vi "Autonomous Independent.vi"() -> ()   [LabVIEW 2017]
doc: "This VI is called when autonomous begins, and will automatically be terminated when autonomous ends. You can carry out timed or sensor driven robot movement independently without needing to return to the caller."
uses:
  <vilib>/Rock Robotics/WPI/Utilities/WPI_GetSetVariantRefNum.vi
  <vilib>/Rock Robotics/Network Tables/NT Write Numeric Array.vi
panel:
  in  "Encoder Input":T1
  out "Rate L 2":dbl
  out "Rate R 2":dbl
  out "Distance L 2":dbl
  out "Direction L 2":bool
  out "Distance R 2":dbl
  out "Direction L 2":bool
  in  "Encoder Input 2":T1
  # "Be sure to right-click and choose Data Operations>>Make Current Value default if you want to save the array values with the VI"
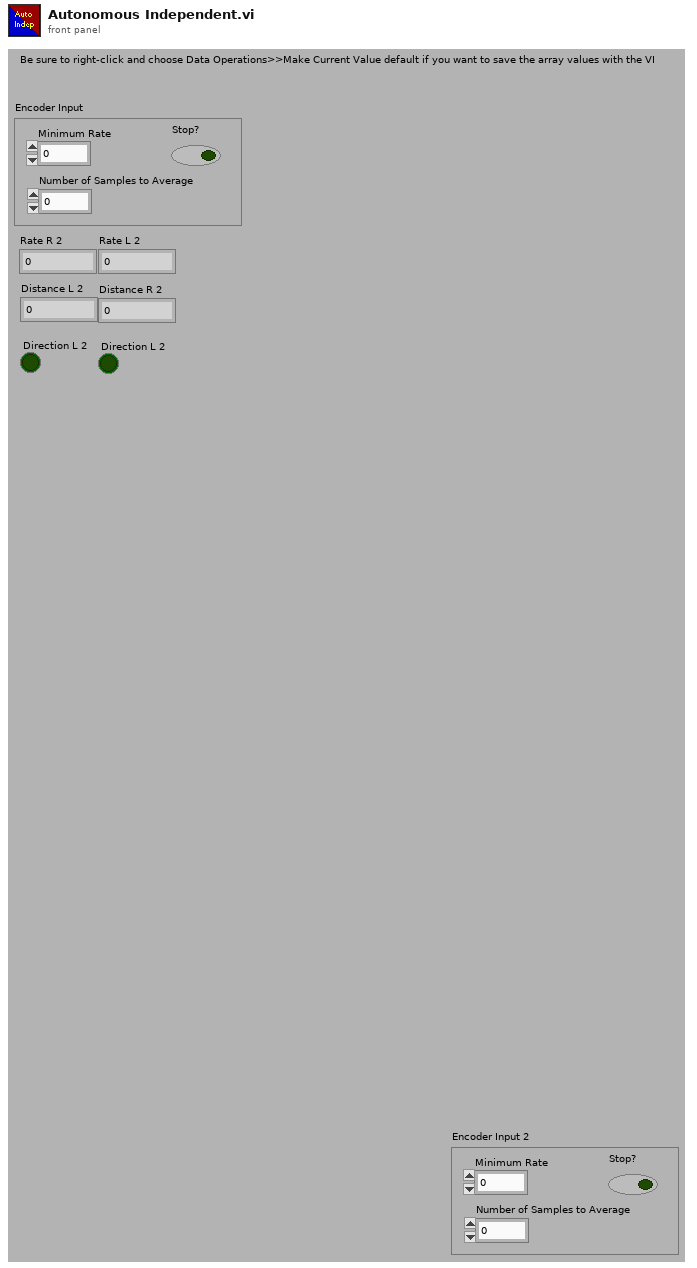
[diagram p1: front panel]
types:
  T1 = cluster{"Minimum Rate":dbl, "Number of Samples to Average":u8, "Stop?":bool}
  T2 = typedef "WPI_JoystickDevRef.ctl" = cluster{"Device":T3}
  T3 = typedef "WPI_JoystickDeviceEnum.ctl" = enum16{"USB 0", "USB 1", "USB 2", "USB 3", "USB 4", "USB 5"}
  T4 = typedef "WPI_RobotDriveDevRef.ctl" = cluster{"DevStatus":errorcluster, "Motors[]":T5[], "Square Inputs":bool, "Max Output":dbl}
  T5 = typedef "WPI_MotorControlDeviceRef.ctl" = cluster{"DeviceStatus":errorcluster, "Type":T6, "PWM":cluster{"PWM Channel":T7, "DeadBand":T8}, "CAN":cluster{"Device Number":u8, "SetOutput VI Ref":variant, "GetOutput VI Ref":variant, "Enable VI Ref":variant, "Disable VI Ref":variant, "Data":variant}, "Invert":bool, "DIO PWM":cluster{"PWM \"Enable\" Channel":T7, "DIOChannel":T9, "PWM Rate":dbl}}
  T6 = typedef "WPI_MotorControlType.ctl" = enum16{"PWM", "CAN", "DIO PWM"}
  T7 = typedef "FPGA_DIOPWMChannel.ctl" = enum8{"PWM 0", "PWM 1", "PWM 2", "PWM 3", "PWM 4", "PWM 5", "PWM 6", "PWM 7", "PWM 8", "PWM 9", "PWM MXP 0", "PWM MXP 1", "PWM MXP 2", "PWM MXP 3", "PWM MXP 4", "PWM MXP 5", "PWM MXP 6", "PWM MXP 7", "PWM MXP 8", "PWM MXP 9", "Invalid"}
  T8 = typedef "WPI_PWMDeadband.ctl" = cluster{"Name":string, "maxPositivePwm":i32, "minPositivePwm":i32, "centerPwm":i32, "maxNegativePwm":i32, "minNegativePwm":i32, "angularRange":u16}
  T9 = typedef "FPGA_DIOChannel.ctl" = enum8{"DIO 0", "DIO 1", "DIO 2", "DIO 3", "DIO 4", "DIO 5", "DIO 6", "DIO 7", "DIO 8", "DIO 9", "DIO MXP 0", "DIO MXP 1", "DIO MXP 2", "DIO MXP 3", "DIO MXP 4", "DIO MXP 5", "DIO MXP 6", "DIO MXP 7", "DIO MXP 8", "DIO MXP 9", "DIO MXP 10", "DIO MXP 11", "DIO MXP 12", "DIO MXP 13", "DIO MXP 14", "DIO MXP 15", "SPI Port CS1", "SPI Port CS2", "SPI Port CS3", "SPI Port MISO", "SPI Port MOSI", "Invalid"}
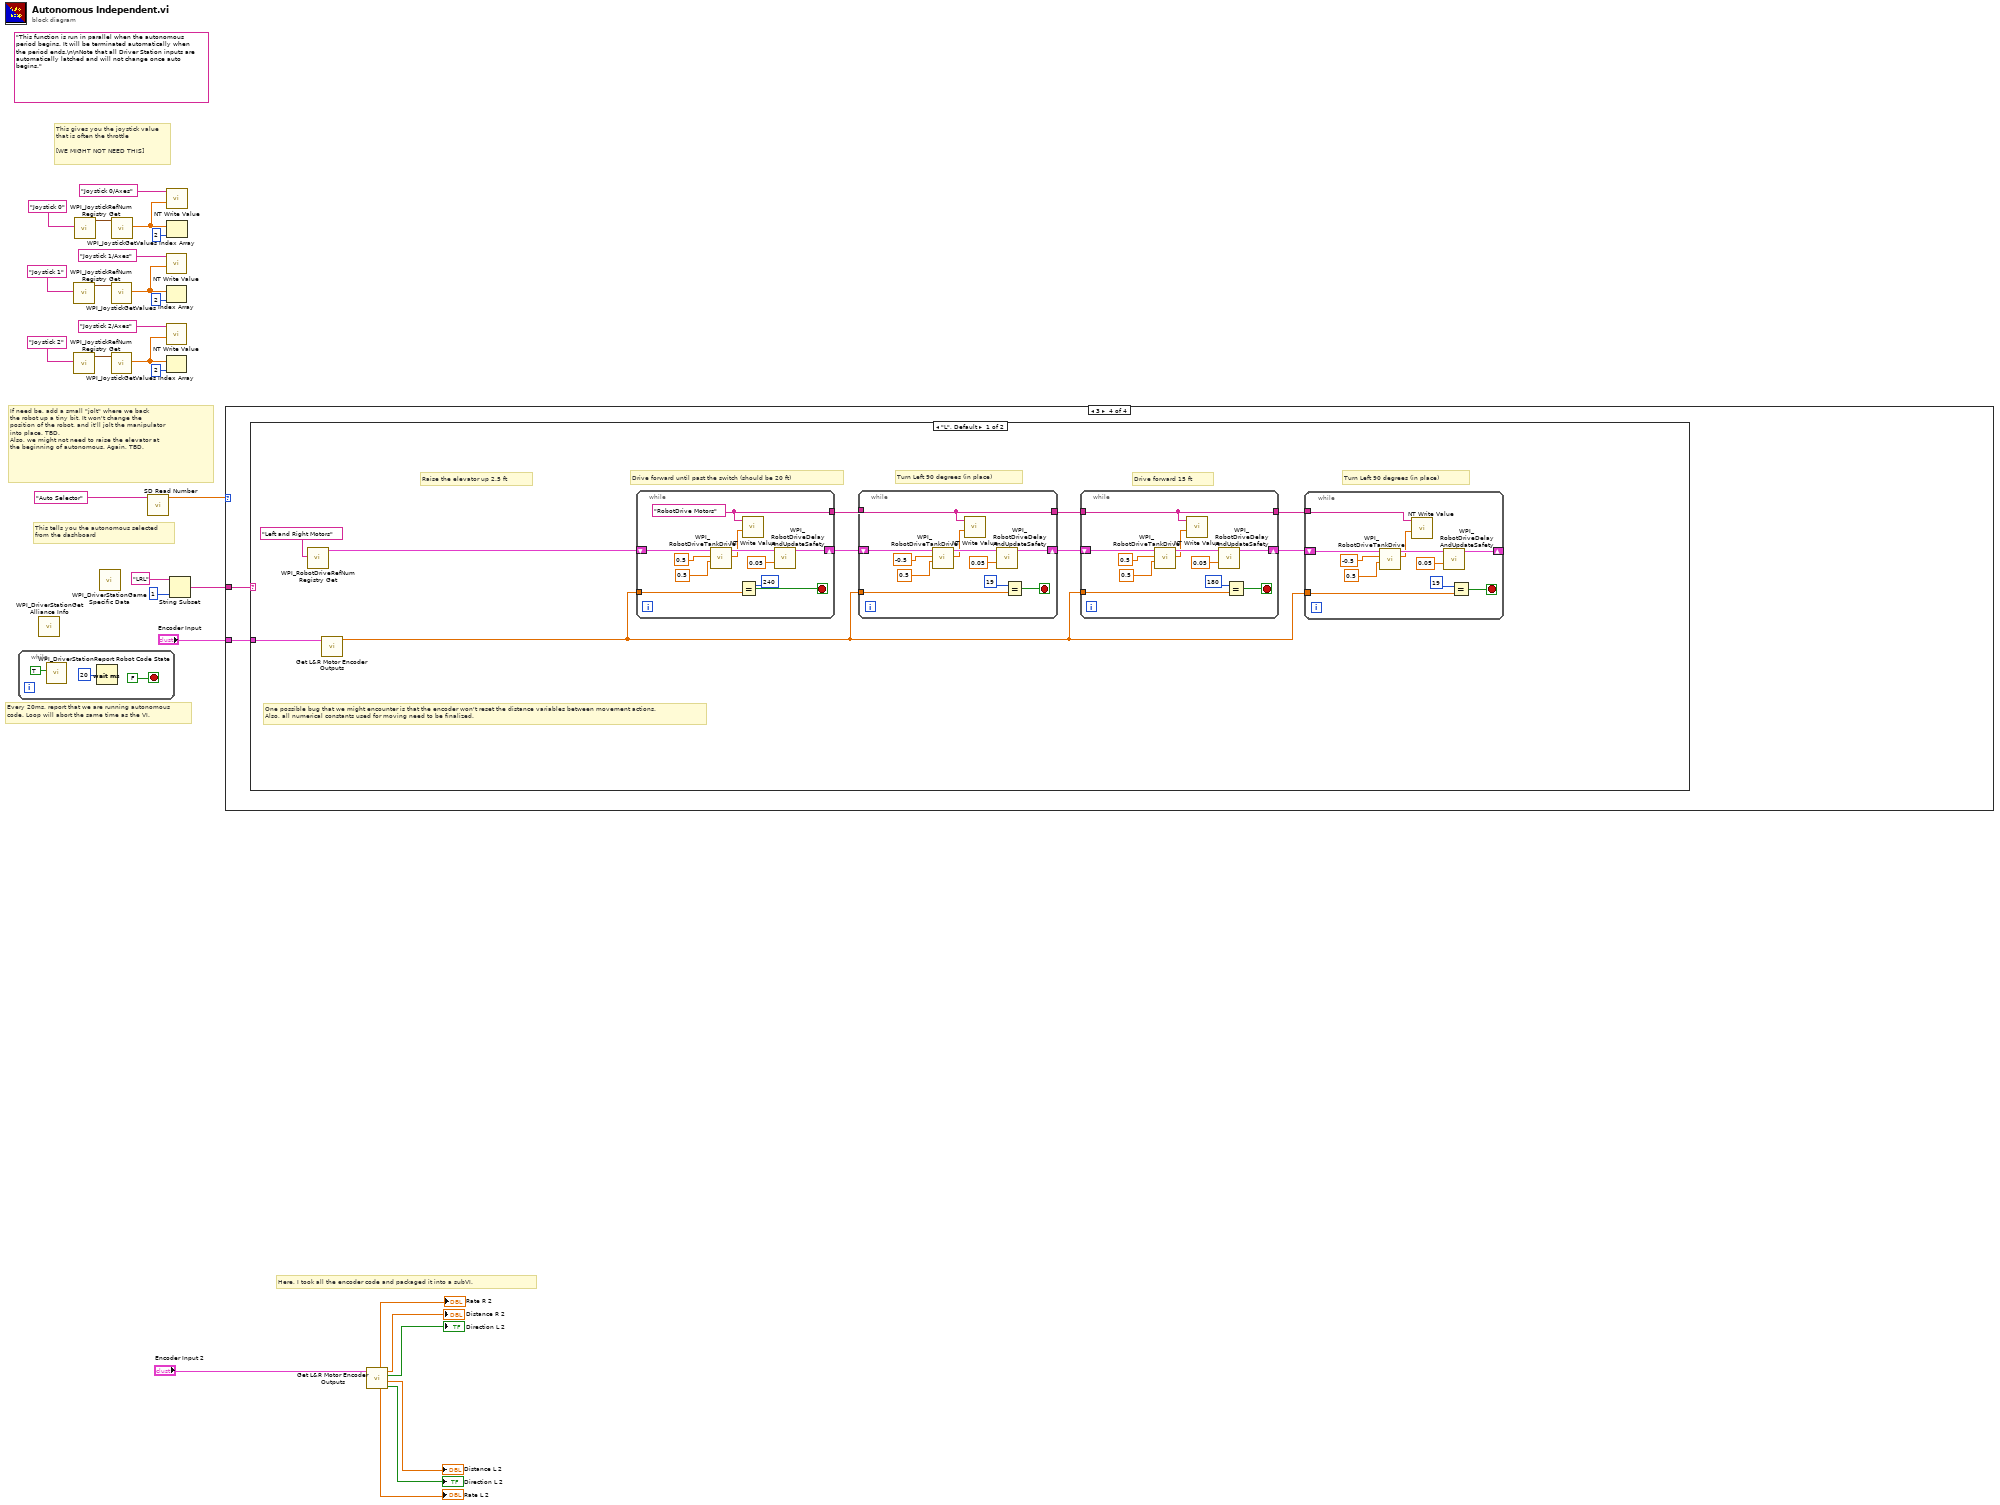
[diagram p0: block diagram]
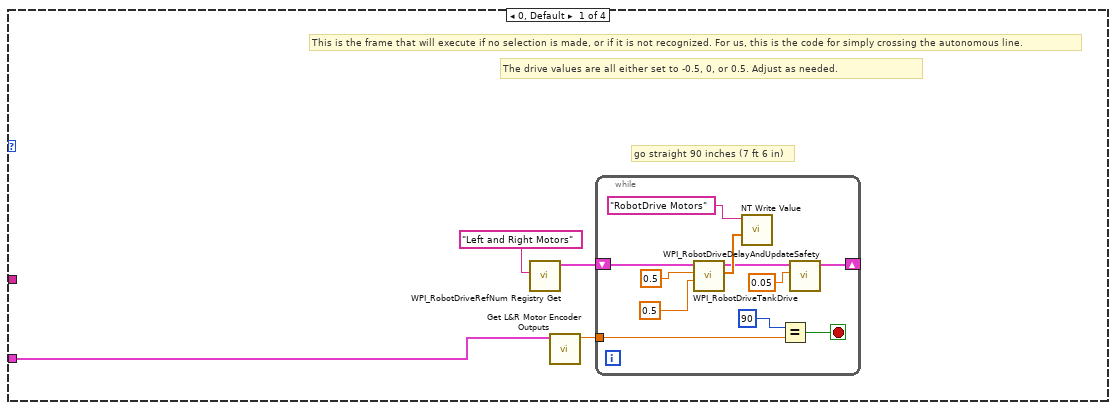
[diagram p2: hidden frame]
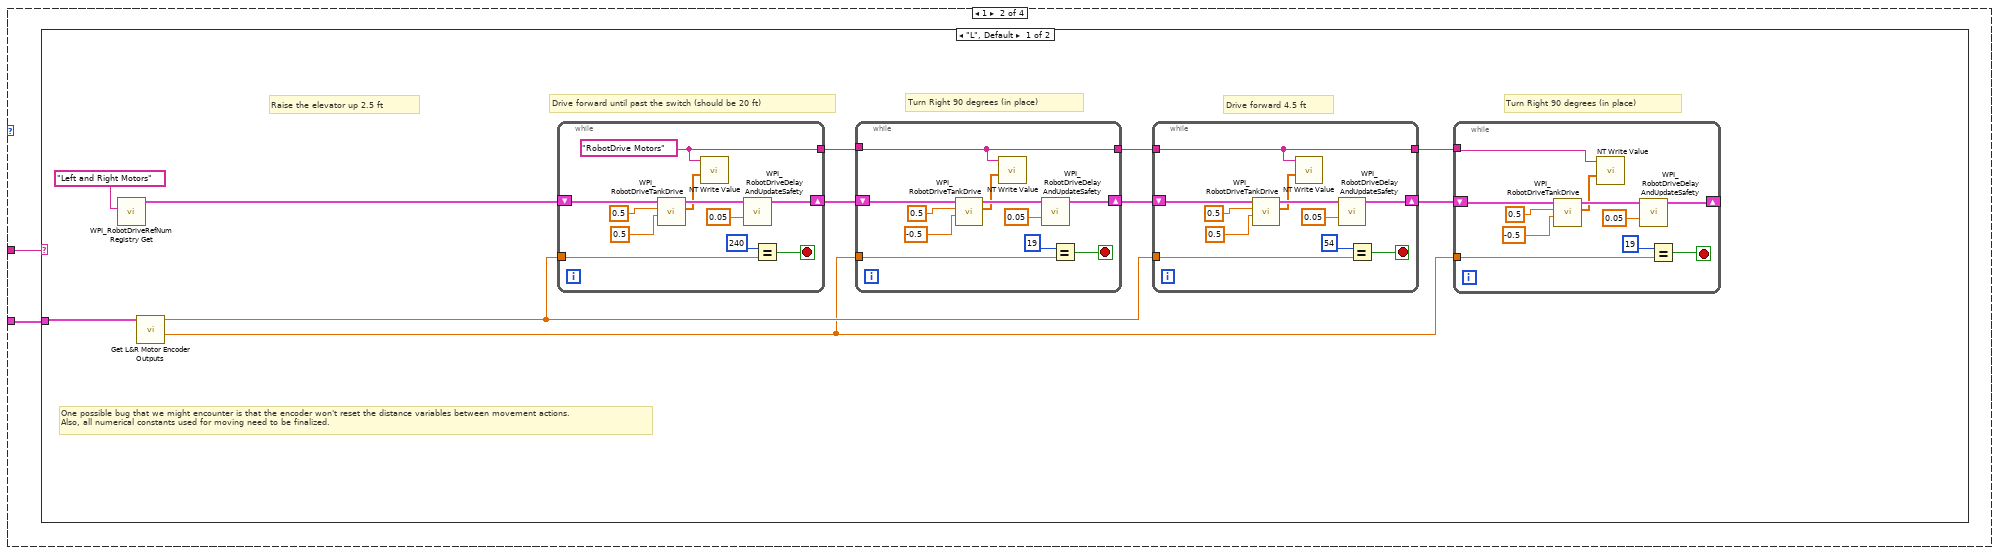
[diagram p3: hidden frame]
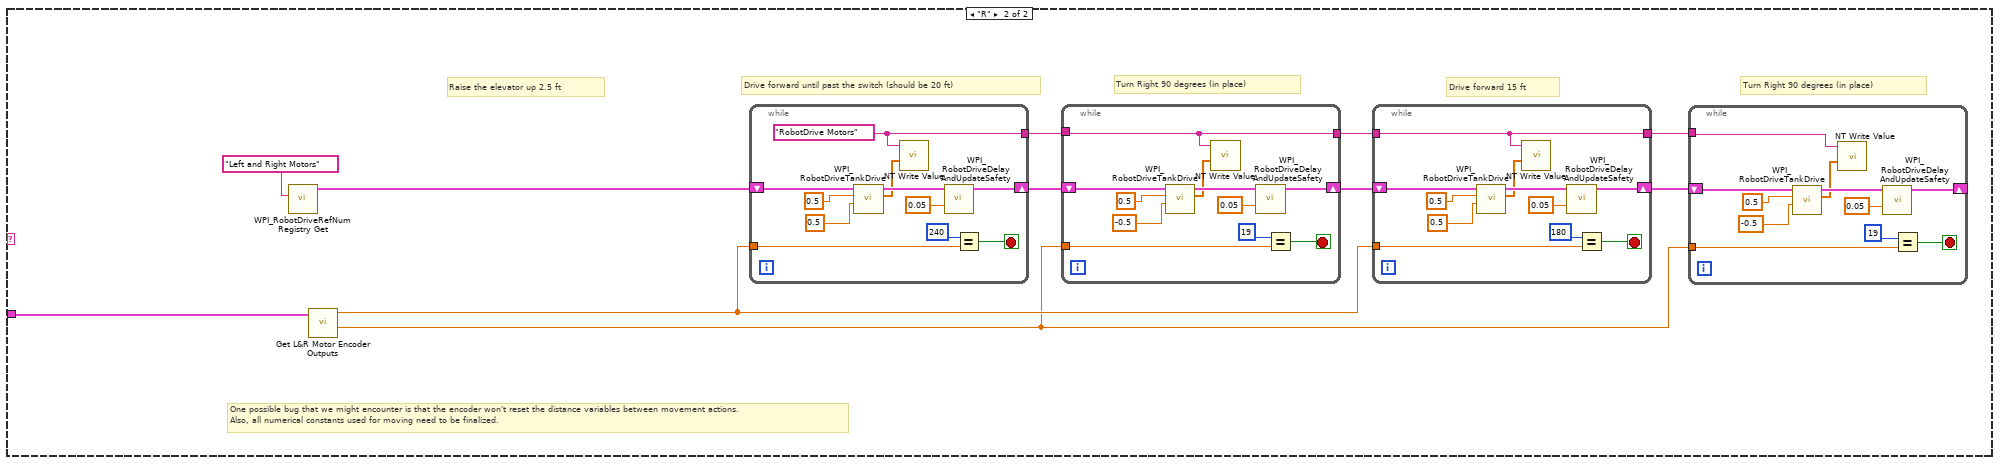
[diagram p4: hidden frame]
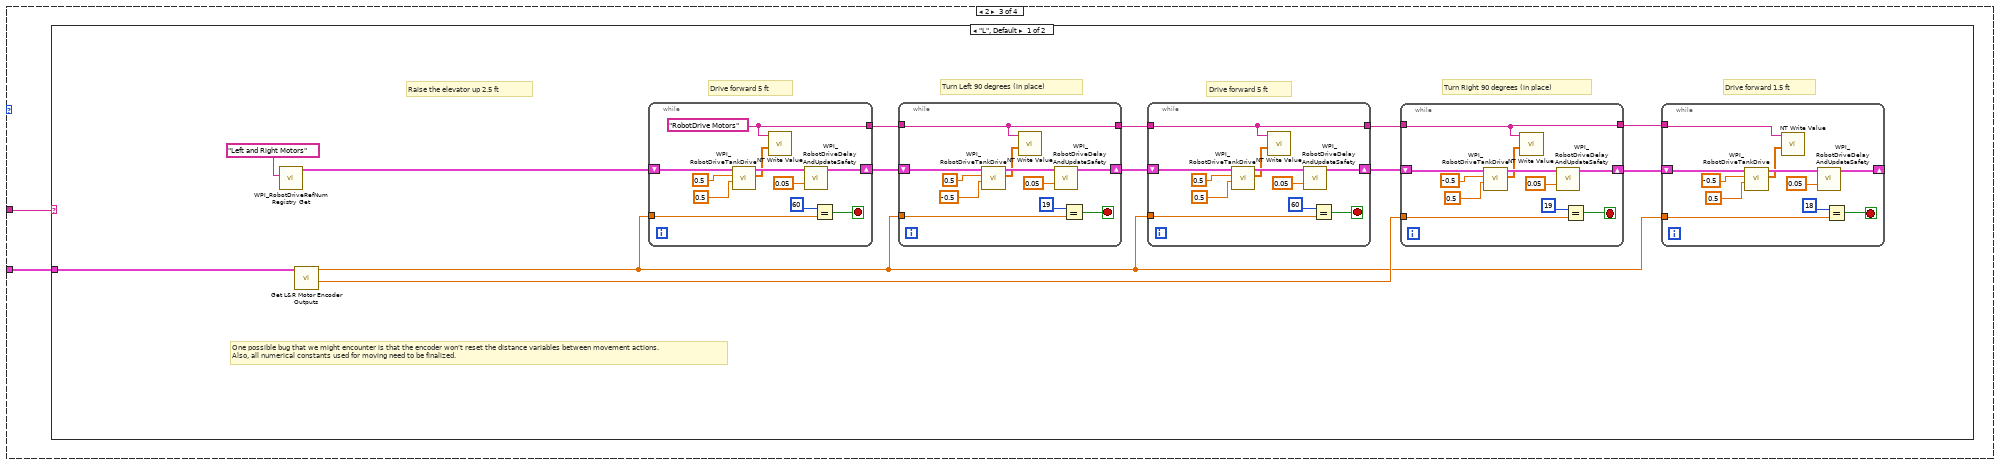
[diagram p5: hidden frame]
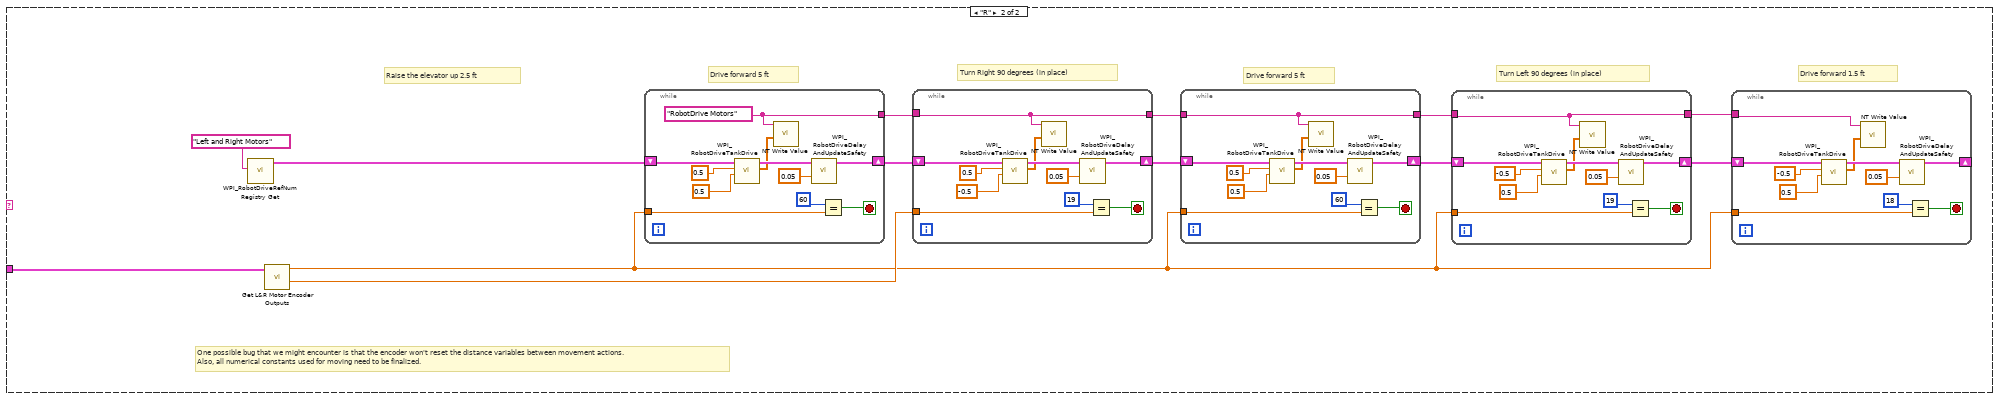
[diagram p6: hidden frame]
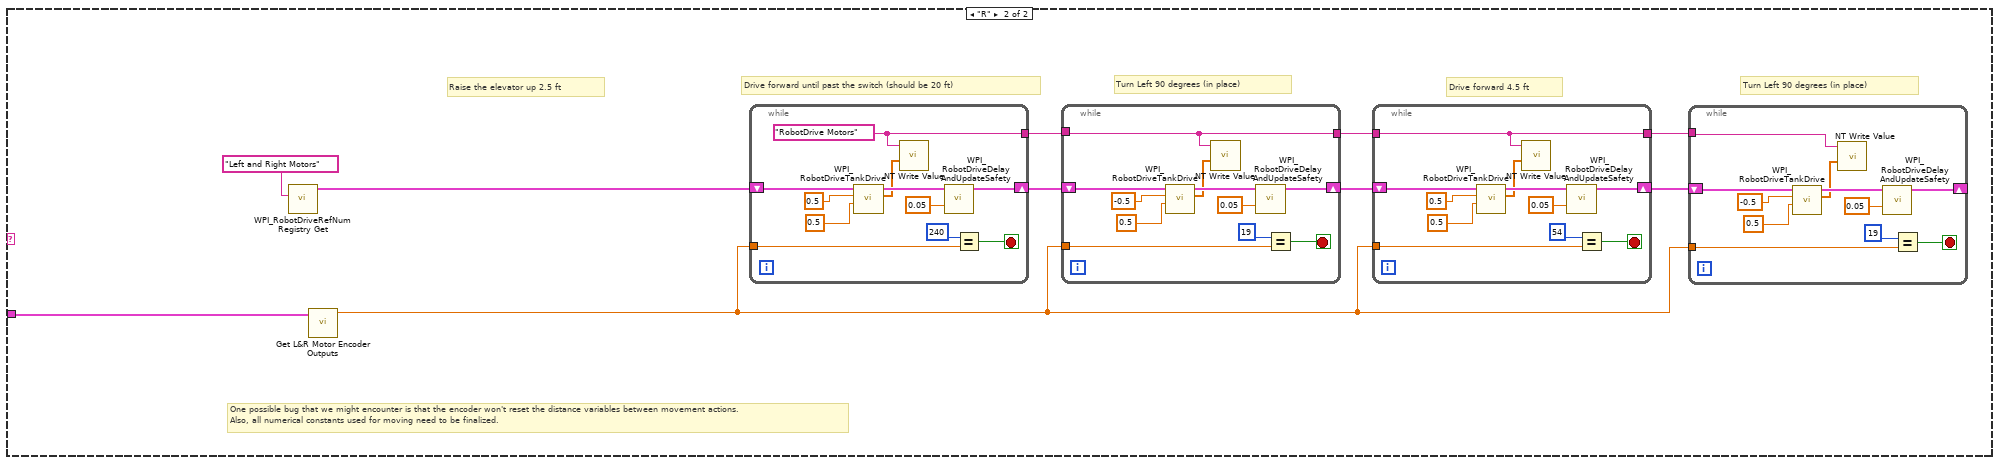
[diagram p7: hidden frame]
diagram:
  (unwired) "This function is run in parallel when the autonomous period begins. It will be terminated automatically when the period ends.\n\nNote that all Driver Station inputs are automatically latched and will not change once auto begins."
  # "If need be, add a small \"jolt\" where we back\nthe robot up a tiny bit. It won't change the\nposition of the robot, and it'll jolt the manipulator\ninto place. TBD.\nAlso, we might not need to raise the elevator at\nthe beginning of autonomous. Again, TBD."
  # "Here, I took all the encoder code and packaged it into a subVI."
  # "This tells you the autonomous selected\nfrom the dashboard"
  # "Every 20ms, report that we are running autonomous\ncode. Loop will abort the same time as the VI."
  # "This gives you the joystick value\nthat is often the throttle\n\n[WE MIGHT NOT NEED THIS]"
  n1 = while {
    stop <- FALSE stop-if-true
    n2 = call <vilib>:"WPI_DriverStationReport Robot Code State.vi"("Autonomous"=TRUE) -> ()  [unwired: 10 in, 1 out]
    n3 = Wait (ms)(milliseconds to wait=u32 20) -> ()  [unwired: 1 out]
  }
  n4 = call <vilib>:"WPI_DriverStationGet Alliance Info.vi"() -> ()  [unwired: 12 out]
  n5 = call <vilib>:"WPI_JoystickRefNum Registry Get.vi"("refnum name"="Joystick 1") -> ("JoystickDevRef"=w22:T2)  [unwired: 1 in, 9 out]
  n6 = call <vilib>:"WPI_JoystickRefNum Registry Get.vi"("refnum name"="Joystick 2") -> ("JoystickDevRef"=w7:T2)  [unwired: 1 in, 9 out]
  n7 = call <vilib>:"WPI_JoystickRefNum Registry Get.vi"("refnum name"="Joystick 0") -> ("JoystickDevRef"=w27:T2)  [unwired: 1 in, 9 out]
  n8 = call <vilib>:"WPI_DriverStationGame Specific Data.vi"() -> ()  [unwired: 11 in, 1 out]
  n9 = call <vilib>:"WPI_JoystickGetValues.vi"("JoystickDevRef"=w22) -> ("Axes"=w20:dbl[])  [unwired: 6 in, 4 out]
  n10 = call <vilib>:"WPI_JoystickGetValues.vi"("JoystickDevRef"=w7) -> ("Axes"=w5:dbl[])  [unwired: 6 in, 4 out]
  n11 = call <vilib>:"WPI_JoystickGetValues.vi"("JoystickDevRef"=w27) -> ("Axes"=w25:dbl[])  [unwired: 6 in, 4 out]
  n12 = call <vilib>:"SD Read Number.vi"("Name"="Auto Selector") -> ("Numeric"=w3:dbl)  [unwired: 8 in, 2 out]
  n13 = call-poly <vilib>:"NT Write Value.vi"("Numeric Array"=w20, "Name"="Joystick 1/Axes") -> ()  [unwired: 9 in, 1 out]
  n14 = Index Array(array=w20, index=2) -> ()  [unwired: 1 out]
  n15 = call-poly <vilib>:"NT Write Value.vi"("Numeric Array"=w5, "Name"="Joystick 2/Axes") -> ()  [unwired: 9 in, 1 out]
  n16 = Index Array(array=w5, index=2) -> ()  [unwired: 1 out]
  n17 = call-poly <vilib>:"NT Write Value.vi"("Numeric Array"=w25, "Name"="Joystick 0/Axes") -> ()  [unwired: 9 in, 1 out]
  n18 = Index Array(array=w25, index=2) -> ()  [unwired: 1 out]
  n19 = String Subset(string="LRL", length (rest)=1) -> (substring=w10:string)  [unwired: 1 in]
  n20 = case shown="3" w3 {
    tunnel: w10 -> [_ w48 w160 w298]
    tunnel: "Encoder Input" -> [w32 w47 w159 w297]
    frame 0, Default {
      # "The drive values are all either set to -0.5, 0, or 0.5. Adjust as needed."
      # "go straight 90 inches (7 ft 6 in)"
      # "This is the frame that will execute if no selection is made, or if it is not recognized. For us, this is the code for simply crossing the autonomous line."
      n21 = call <vilib>:"WPI_RobotDriveRefNum Registry Get.vi"("refnum name"="Left and Right Motors") -> ("RobotDriveDevRef"=w34:T4)  [unwired: 1 in, 9 out]
      n22 = call <vilib>:"Get L&R Motor Encoder Outputs.vi"("Encoder Input in"=w32) -> ("Distance R"=w33:dbl)  [unwired: 5 in, 5 out]
      n23 = while {
        shift-right: [w38] -> _
        shift-left: w34 -> [w43]
        tunnel: w33 -> [w36]
        stop <- w37 stop-if-true
        n24 = call <vilib>:"WPI_RobotDriveTankDrive.vi"("Right axis value"=0.5 ("X axis value"), "Left axis value"=0.5 ("X axis value"), "RobotDriveDevRef"=w43) -> ("Motor Values"=w46:dbl[], "RobotDriveDevRef"=w39:T4)  [unwired: 6 in, 1 out]
        n25 = call-poly <vilib>:"NT Write Value.vi"("Numeric Array"=w46, "Name"="RobotDrive Motors") -> ()  [unwired: 9 in, 1 out]
        n26 = Equal?(x=90, y=w36) -> (x = y?=w37:bool)
        n27 = call <vilib>:"WPI_RobotDriveDelayAndUpdateSafety.vi"("Delay (s)"=0.05, "RobotDriveDevRef"=w39) -> ("RobotDriveDevRef 2"=w38:T4)  [unwired: 8 in, 1 out]
      }
    }
    frame 1 {
      n28 = case shown="\"L\", Default" w48 {
        tunnel: w47 -> [w49 w104]
        frame "L", Default {
          # "Raise the elevator up 2.5 ft"
          # "Turn Right 90 degrees (in place)"
          # "Drive forward 4.5 ft"
          # "One possible bug that we might encounter is that the encoder won't reset the distance variables between movement actions.\nAlso, all numerical constants used for moving need to be finalized."
          # "Turn Right 90 degrees (in place)"
          # "Drive forward until past the switch (should be 20 ft)"
          n29 = call <vilib>:"WPI_RobotDriveRefNum Registry Get.vi"("refnum name"="Left and Right Motors") -> ("RobotDriveDevRef"=w58:T4)  [unwired: 1 in, 9 out]
          n30 = call <vilib>:"Get L&R Motor Encoder Outputs.vi"("Encoder Input in"=w49) -> ("Distance L"=w50:dbl, "Distance R"=w53:dbl)  [unwired: 5 in, 4 out]
          n31 = while {
            tunnel: w53 -> [w102]
            shift-right: [w97] -> w57
            shift-left: w58 -> [w98]
            tunnel: [w96] -> w56
            stop <- w103 stop-if-true
            w96 = "RobotDrive Motors" ("Name")
            n32 = call <vilib>:"WPI_RobotDriveTankDrive.vi"("Right axis value"=0.5 ("X axis value"), "Left axis value"=0.5 ("X axis value"), "RobotDriveDevRef"=w98) -> ("Motor Values"=w100:dbl[], "RobotDriveDevRef"=w101:T4)  [unwired: 6 in, 1 out]
            n33 = call-poly <vilib>:"NT Write Value.vi"("Numeric Array"=w100, "Name"=w96) -> ()  [unwired: 9 in, 1 out]
            n34 = call <vilib>:"WPI_RobotDriveDelayAndUpdateSafety.vi"("Delay (s)"=0.05, "RobotDriveDevRef"=w101) -> ("RobotDriveDevRef 2"=w97:T4)  [unwired: 8 in, 1 out]
            n35 = Equal?(x=240, y=w102) -> (x = y?=w103:bool)
          }
          n36 = while {
            shift-right: [w87] -> w54
            shift-left: w57 -> [w88]
            tunnel: [w83] -> w55
            tunnel: w56 -> [w83]
            tunnel: w50 -> [w82]
            stop <- w92 stop-if-true
            n37 = call <vilib>:"WPI_RobotDriveTankDrive.vi"("Right axis value"=-0.5 ("X axis value"), "Left axis value"=0.5 ("X axis value"), "RobotDriveDevRef"=w88) -> ("Motor Values"=w90:dbl[], "RobotDriveDevRef"=w91:T4)  [unwired: 6 in, 1 out]
            n38 = call-poly <vilib>:"NT Write Value.vi"("Numeric Array"=w90, "Name"=w83) -> ()  [unwired: 9 in, 1 out]
            n39 = call <vilib>:"WPI_RobotDriveDelayAndUpdateSafety.vi"("Delay (s)"=0.05, "RobotDriveDevRef"=w91) -> ("RobotDriveDevRef 2"=w87:T4)  [unwired: 8 in, 1 out]
            n40 = Equal?(x=19, y=w82) -> (x = y?=w92:bool)
          }
          n41 = while {
            tunnel: w53 -> [w80]
            shift-right: [w75] -> w51
            shift-left: w54 -> [w76]
            tunnel: [w71] -> w52
            tunnel: w55 -> [w71]
            stop <- w81 stop-if-true
            n42 = call <vilib>:"WPI_RobotDriveTankDrive.vi"("Right axis value"=0.5 ("X axis value"), "Left axis value"=0.5 ("X axis value"), "RobotDriveDevRef"=w76) -> ("Motor Values"=w78:dbl[], "RobotDriveDevRef"=w79:T4)  [unwired: 6 in, 1 out]
            n43 = call-poly <vilib>:"NT Write Value.vi"("Numeric Array"=w78, "Name"=w71) -> ()  [unwired: 9 in, 1 out]
            n44 = call <vilib>:"WPI_RobotDriveDelayAndUpdateSafety.vi"("Delay (s)"=0.05, "RobotDriveDevRef"=w79) -> ("RobotDriveDevRef 2"=w75:T4)  [unwired: 8 in, 1 out]
            n45 = Equal?(x=54, y=w80) -> (x = y?=w81:bool)
          }
          n46 = while {
            shift-right: [w65] -> _
            shift-left: w51 -> [w66]
            tunnel: w52 -> [w61]
            tunnel: w50 -> [w60]
            stop <- w70 stop-if-true
            n47 = call <vilib>:"WPI_RobotDriveTankDrive.vi"("Right axis value"=-0.5 ("X axis value"), "Left axis value"=0.5 ("X axis value"), "RobotDriveDevRef"=w66) -> ("Motor Values"=w68:dbl[], "RobotDriveDevRef"=w69:T4)  [unwired: 6 in, 1 out]
            n48 = call-poly <vilib>:"NT Write Value.vi"("Numeric Array"=w68, "Name"=w61) -> ()  [unwired: 9 in, 1 out]
            n49 = call <vilib>:"WPI_RobotDriveDelayAndUpdateSafety.vi"("Delay (s)"=0.05, "RobotDriveDevRef"=w69) -> ("RobotDriveDevRef 2"=w65:T4)  [unwired: 8 in, 1 out]
            n50 = Equal?(x=19, y=w60) -> (x = y?=w70:bool)
          }
        }
        frame "R" {
          # "Raise the elevator up 2.5 ft"
          # "Turn Right 90 degrees (in place)"
          # "Drive forward 15 ft"
          # "One possible bug that we might encounter is that the encoder won't reset the distance variables between movement actions.\nAlso, all numerical constants used for moving need to be finalized."
          # "Turn Right 90 degrees (in place)"
          # "Drive forward until past the switch (should be 20 ft)"
          n51 = call <vilib>:"WPI_RobotDriveRefNum Registry Get.vi"("refnum name"="Left and Right Motors") -> ("RobotDriveDevRef"=w113:T4)  [unwired: 1 in, 9 out]
          n52 = call <vilib>:"Get L&R Motor Encoder Outputs.vi"("Encoder Input in"=w104) -> ("Distance L"=w105:dbl, "Distance R"=w108:dbl)  [unwired: 5 in, 4 out]
          n53 = while {
            tunnel: w108 -> [w157]
            shift-right: [w152] -> w112
            shift-left: w113 -> [w153]
            tunnel: [w151] -> w111
            stop <- w158 stop-if-true
            w151 = "RobotDrive Motors" ("Name")
            n54 = call <vilib>:"WPI_RobotDriveTankDrive.vi"("Right axis value"=0.5 ("X axis value"), "Left axis value"=0.5 ("X axis value"), "RobotDriveDevRef"=w153) -> ("Motor Values"=w155:dbl[], "RobotDriveDevRef"=w156:T4)  [unwired: 6 in, 1 out]
            n55 = call-poly <vilib>:"NT Write Value.vi"("Numeric Array"=w155, "Name"=w151) -> ()  [unwired: 9 in, 1 out]
            n56 = call <vilib>:"WPI_RobotDriveDelayAndUpdateSafety.vi"("Delay (s)"=0.05, "RobotDriveDevRef"=w156) -> ("RobotDriveDevRef 2"=w152:T4)  [unwired: 8 in, 1 out]
            n57 = Equal?(x=240, y=w157) -> (x = y?=w158:bool)
          }
          n58 = while {
            shift-right: [w142] -> w109
            shift-left: w112 -> [w143]
            tunnel: [w138] -> w110
            tunnel: w111 -> [w138]
            tunnel: w105 -> [w137]
            stop <- w147 stop-if-true
            n59 = call <vilib>:"WPI_RobotDriveTankDrive.vi"("Right axis value"=-0.5 ("X axis value"), "Left axis value"=0.5 ("X axis value"), "RobotDriveDevRef"=w143) -> ("Motor Values"=w145:dbl[], "RobotDriveDevRef"=w146:T4)  [unwired: 6 in, 1 out]
            n60 = call-poly <vilib>:"NT Write Value.vi"("Numeric Array"=w145, "Name"=w138) -> ()  [unwired: 9 in, 1 out]
            n61 = call <vilib>:"WPI_RobotDriveDelayAndUpdateSafety.vi"("Delay (s)"=0.05, "RobotDriveDevRef"=w146) -> ("RobotDriveDevRef 2"=w142:T4)  [unwired: 8 in, 1 out]
            n62 = Equal?(x=19, y=w137) -> (x = y?=w147:bool)
          }
          n63 = while {
            tunnel: w108 -> [w135]
            shift-right: [w130] -> w106
            shift-left: w109 -> [w131]
            tunnel: [w126] -> w107
            tunnel: w110 -> [w126]
            stop <- w136 stop-if-true
            n64 = call <vilib>:"WPI_RobotDriveTankDrive.vi"("Right axis value"=0.5 ("X axis value"), "Left axis value"=0.5 ("X axis value"), "RobotDriveDevRef"=w131) -> ("Motor Values"=w133:dbl[], "RobotDriveDevRef"=w134:T4)  [unwired: 6 in, 1 out]
            n65 = call-poly <vilib>:"NT Write Value.vi"("Numeric Array"=w133, "Name"=w126) -> ()  [unwired: 9 in, 1 out]
            n66 = call <vilib>:"WPI_RobotDriveDelayAndUpdateSafety.vi"("Delay (s)"=0.05, "RobotDriveDevRef"=w134) -> ("RobotDriveDevRef 2"=w130:T4)  [unwired: 8 in, 1 out]
            n67 = Equal?(x=180, y=w135) -> (x = y?=w136:bool)
          }
          n68 = while {
            shift-right: [w120] -> _
            shift-left: w106 -> [w121]
            tunnel: w107 -> [w116]
            tunnel: w105 -> [w115]
            stop <- w125 stop-if-true
            n69 = call <vilib>:"WPI_RobotDriveTankDrive.vi"("Right axis value"=-0.5 ("X axis value"), "Left axis value"=0.5 ("X axis value"), "RobotDriveDevRef"=w121) -> ("Motor Values"=w123:dbl[], "RobotDriveDevRef"=w124:T4)  [unwired: 6 in, 1 out]
            n70 = call-poly <vilib>:"NT Write Value.vi"("Numeric Array"=w123, "Name"=w116) -> ()  [unwired: 9 in, 1 out]
            n71 = call <vilib>:"WPI_RobotDriveDelayAndUpdateSafety.vi"("Delay (s)"=0.05, "RobotDriveDevRef"=w124) -> ("RobotDriveDevRef 2"=w120:T4)  [unwired: 8 in, 1 out]
            n72 = Equal?(x=19, y=w115) -> (x = y?=w125:bool)
          }
        }
      }
    }
    frame 2 {
      n73 = case shown="\"L\", Default" w160 {
        tunnel: w159 -> [w163 w232]
        frame "L", Default {
          # "Drive forward 1.5 ft"
          # "Raise the elevator up 2.5 ft"
          # "Turn Right 90 degrees (in place)"
          # "Drive forward 5 ft"
          # "One possible bug that we might encounter is that the encoder won't reset the distance variables between movement actions.\nAlso, all numerical constants used for moving need to be finalized."
          # "Turn Left 90 degrees (in place)"
          # "Drive forward 5 ft"
          n74 = call <vilib>:"WPI_RobotDriveRefNum Registry Get.vi"("refnum name"="Left and Right Motors") -> ("RobotDriveDevRef"=w165:T4)  [unwired: 1 in, 9 out]
          n75 = call <vilib>:"Get L&R Motor Encoder Outputs.vi"("Encoder Input in"=w163) -> ("Distance L"=w162:dbl, "Distance R"=w161:dbl)  [unwired: 5 in, 4 out]
          n76 = while {
            tunnel: w161 -> [w227]
            shift-right: [w222] -> w166
            shift-left: w165 -> [w223]
            tunnel: [w221] -> w167
            stop <- w228 stop-if-true
            w221 = "RobotDrive Motors" ("Name")
            n77 = call <vilib>:"WPI_RobotDriveTankDrive.vi"("Right axis value"=0.5 ("X axis value"), "Left axis value"=0.5 ("X axis value"), "RobotDriveDevRef"=w223) -> ("Motor Values"=w225:dbl[], "RobotDriveDevRef"=w226:T4)  [unwired: 6 in, 1 out]
            n78 = call-poly <vilib>:"NT Write Value.vi"("Numeric Array"=w225, "Name"=w221) -> ()  [unwired: 9 in, 1 out]
            n79 = call <vilib>:"WPI_RobotDriveDelayAndUpdateSafety.vi"("Delay (s)"=0.05, "RobotDriveDevRef"=w226) -> ("RobotDriveDevRef 2"=w222:T4)  [unwired: 8 in, 1 out]
            n80 = Equal?(x=60, y=w227) -> (x = y?=w228:bool)
          }
          n81 = while {
            shift-right: [w212] -> w169
            shift-left: w166 -> [w213]
            tunnel: [w208] -> w168
            tunnel: w167 -> [w208]
            tunnel: w161 -> [w207]
            stop <- w217 stop-if-true
            n82 = call <vilib>:"WPI_RobotDriveTankDrive.vi"("Right axis value"=-0.5 ("X axis value"), "Left axis value"=0.5 ("X axis value"), "RobotDriveDevRef"=w213) -> ("Motor Values"=w215:dbl[], "RobotDriveDevRef"=w216:T4)  [unwired: 6 in, 1 out]
            n83 = call-poly <vilib>:"NT Write Value.vi"("Numeric Array"=w215, "Name"=w208) -> ()  [unwired: 9 in, 1 out]
            n84 = call <vilib>:"WPI_RobotDriveDelayAndUpdateSafety.vi"("Delay (s)"=0.05, "RobotDriveDevRef"=w216) -> ("RobotDriveDevRef 2"=w212:T4)  [unwired: 8 in, 1 out]
            n85 = Equal?(x=19, y=w207) -> (x = y?=w217:bool)
          }
          n86 = while {
            tunnel: w161 -> [w205]
            shift-right: [w200] -> w171
            shift-left: w169 -> [w201]
            tunnel: [w196] -> w170
            tunnel: w168 -> [w196]
            stop <- w206 stop-if-true
            n87 = call <vilib>:"WPI_RobotDriveTankDrive.vi"("Right axis value"=0.5 ("X axis value"), "Left axis value"=0.5 ("X axis value"), "RobotDriveDevRef"=w201) -> ("Motor Values"=w203:dbl[], "RobotDriveDevRef"=w204:T4)  [unwired: 6 in, 1 out]
            n88 = call-poly <vilib>:"NT Write Value.vi"("Numeric Array"=w203, "Name"=w196) -> ()  [unwired: 9 in, 1 out]
            n89 = call <vilib>:"WPI_RobotDriveDelayAndUpdateSafety.vi"("Delay (s)"=0.05, "RobotDriveDevRef"=w204) -> ("RobotDriveDevRef 2"=w200:T4)  [unwired: 8 in, 1 out]
            n90 = Equal?(x=60, y=w205) -> (x = y?=w206:bool)
          }
          n91 = while {
            shift-right: [w190] -> w172
            shift-left: w171 -> [w191]
            tunnel: w170 -> [w185]
            tunnel: w162 -> [w186]
            tunnel: [w185] -> w173
            stop <- w195 stop-if-true
            n92 = call <vilib>:"WPI_RobotDriveTankDrive.vi"("Right axis value"=0.5 ("X axis value"), "Left axis value"=-0.5 ("X axis value"), "RobotDriveDevRef"=w191) -> ("Motor Values"=w193:dbl[], "RobotDriveDevRef"=w194:T4)  [unwired: 6 in, 1 out]
            n93 = call-poly <vilib>:"NT Write Value.vi"("Numeric Array"=w193, "Name"=w185) -> ()  [unwired: 9 in, 1 out]
            n94 = call <vilib>:"WPI_RobotDriveDelayAndUpdateSafety.vi"("Delay (s)"=0.05, "RobotDriveDevRef"=w194) -> ("RobotDriveDevRef 2"=w190:T4)  [unwired: 8 in, 1 out]
            n95 = Equal?(x=19, y=w186) -> (x = y?=w195:bool)
          }
          n96 = while {
            shift-right: [w179] -> _
            shift-left: w172 -> [w180]
            tunnel: w173 -> [w175]
            tunnel: w161 -> [w174]
            stop <- w184 stop-if-true
            n97 = call <vilib>:"WPI_RobotDriveTankDrive.vi"("Right axis value"=0.5 ("X axis value"), "Left axis value"=-0.5 ("X axis value"), "RobotDriveDevRef"=w180) -> ("Motor Values"=w182:dbl[], "RobotDriveDevRef"=w183:T4)  [unwired: 6 in, 1 out]
            n98 = call-poly <vilib>:"NT Write Value.vi"("Numeric Array"=w182, "Name"=w175) -> ()  [unwired: 9 in, 1 out]
            n99 = call <vilib>:"WPI_RobotDriveDelayAndUpdateSafety.vi"("Delay (s)"=0.05, "RobotDriveDevRef"=w183) -> ("RobotDriveDevRef 2"=w179:T4)  [unwired: 8 in, 1 out]
            n100 = Equal?(x=18, y=w174) -> (x = y?=w184:bool)
          }
        }
        frame "R" {
          # "Drive forward 1.5 ft"
          # "Raise the elevator up 2.5 ft"
          # "Turn Left 90 degrees (in place)"
          # "Drive forward 5 ft"
          # "One possible bug that we might encounter is that the encoder won't reset the distance variables between movement actions.\nAlso, all numerical constants used for moving need to be finalized."
          # "Turn Right 90 degrees (in place)"
          # "Drive forward 5 ft"
          n101 = call <vilib>:"WPI_RobotDriveRefNum Registry Get.vi"("refnum name"="Left and Right Motors") -> ("RobotDriveDevRef"=w240:T4)  [unwired: 1 in, 9 out]
          n102 = call <vilib>:"Get L&R Motor Encoder Outputs.vi"("Encoder Input in"=w232) -> ("Distance L"=w233:dbl, "Distance R"=w229:dbl)  [unwired: 5 in, 4 out]
          n103 = while {
            tunnel: w229 -> [w295]
            shift-right: [w290] -> w239
            shift-left: w240 -> [w291]
            tunnel: [w289] -> w238
            stop <- w296 stop-if-true
            w289 = "RobotDrive Motors" ("Name")
            n104 = call <vilib>:"WPI_RobotDriveTankDrive.vi"("Right axis value"=0.5 ("X axis value"), "Left axis value"=0.5 ("X axis value"), "RobotDriveDevRef"=w291) -> ("Motor Values"=w293:dbl[], "RobotDriveDevRef"=w294:T4)  [unwired: 6 in, 1 out]
            n105 = call-poly <vilib>:"NT Write Value.vi"("Numeric Array"=w293, "Name"=w289) -> ()  [unwired: 9 in, 1 out]
            n106 = call <vilib>:"WPI_RobotDriveDelayAndUpdateSafety.vi"("Delay (s)"=0.05, "RobotDriveDevRef"=w294) -> ("RobotDriveDevRef 2"=w290:T4)  [unwired: 8 in, 1 out]
            n107 = Equal?(x=60, y=w295) -> (x = y?=w296:bool)
          }
          n108 = while {
            shift-right: [w280] -> w236
            shift-left: w239 -> [w281]
            tunnel: [w276] -> w237
            tunnel: w238 -> [w276]
            tunnel: w233 -> [w275]
            stop <- w285 stop-if-true
            n109 = call <vilib>:"WPI_RobotDriveTankDrive.vi"("Right axis value"=-0.5 ("X axis value"), "Left axis value"=0.5 ("X axis value"), "RobotDriveDevRef"=w281) -> ("Motor Values"=w283:dbl[], "RobotDriveDevRef"=w284:T4)  [unwired: 6 in, 1 out]
            n110 = call-poly <vilib>:"NT Write Value.vi"("Numeric Array"=w283, "Name"=w276) -> ()  [unwired: 9 in, 1 out]
            n111 = call <vilib>:"WPI_RobotDriveDelayAndUpdateSafety.vi"("Delay (s)"=0.05, "RobotDriveDevRef"=w284) -> ("RobotDriveDevRef 2"=w280:T4)  [unwired: 8 in, 1 out]
            n112 = Equal?(x=19, y=w275) -> (x = y?=w285:bool)
          }
          n113 = while {
            tunnel: w229 -> [w273]
            shift-right: [w268] -> w234
            shift-left: w236 -> [w269]
            tunnel: [w264] -> w235
            tunnel: w237 -> [w264]
            stop <- w274 stop-if-true
            n114 = call <vilib>:"WPI_RobotDriveTankDrive.vi"("Right axis value"=0.5 ("X axis value"), "Left axis value"=0.5 ("X axis value"), "RobotDriveDevRef"=w269) -> ("Motor Values"=w271:dbl[], "RobotDriveDevRef"=w272:T4)  [unwired: 6 in, 1 out]
            n115 = call-poly <vilib>:"NT Write Value.vi"("Numeric Array"=w271, "Name"=w264) -> ()  [unwired: 9 in, 1 out]
            n116 = call <vilib>:"WPI_RobotDriveDelayAndUpdateSafety.vi"("Delay (s)"=0.05, "RobotDriveDevRef"=w272) -> ("RobotDriveDevRef 2"=w268:T4)  [unwired: 8 in, 1 out]
            n117 = Equal?(x=60, y=w273) -> (x = y?=w274:bool)
          }
          n118 = while {
            shift-right: [w258] -> w231
            shift-left: w234 -> [w259]
            tunnel: w235 -> [w253]
            tunnel: w229 -> [w254]
            tunnel: [w253] -> w230
            stop <- w263 stop-if-true
            n119 = call <vilib>:"WPI_RobotDriveTankDrive.vi"("Right axis value"=0.5 ("X axis value"), "Left axis value"=-0.5 ("X axis value"), "RobotDriveDevRef"=w259) -> ("Motor Values"=w261:dbl[], "RobotDriveDevRef"=w262:T4)  [unwired: 6 in, 1 out]
            n120 = call-poly <vilib>:"NT Write Value.vi"("Numeric Array"=w261, "Name"=w253) -> ()  [unwired: 9 in, 1 out]
            n121 = call <vilib>:"WPI_RobotDriveDelayAndUpdateSafety.vi"("Delay (s)"=0.05, "RobotDriveDevRef"=w262) -> ("RobotDriveDevRef 2"=w258:T4)  [unwired: 8 in, 1 out]
            n122 = Equal?(x=19, y=w254) -> (x = y?=w263:bool)
          }
          n123 = while {
            shift-right: [w247] -> _
            shift-left: w231 -> [w248]
            tunnel: w230 -> [w243]
            tunnel: w229 -> [w242]
            stop <- w252 stop-if-true
            n124 = call <vilib>:"WPI_RobotDriveTankDrive.vi"("Right axis value"=0.5 ("X axis value"), "Left axis value"=-0.5 ("X axis value"), "RobotDriveDevRef"=w248) -> ("Motor Values"=w250:dbl[], "RobotDriveDevRef"=w251:T4)  [unwired: 6 in, 1 out]
            n125 = call-poly <vilib>:"NT Write Value.vi"("Numeric Array"=w250, "Name"=w243) -> ()  [unwired: 9 in, 1 out]
            n126 = call <vilib>:"WPI_RobotDriveDelayAndUpdateSafety.vi"("Delay (s)"=0.05, "RobotDriveDevRef"=w251) -> ("RobotDriveDevRef 2"=w247:T4)  [unwired: 8 in, 1 out]
            n127 = Equal?(x=18, y=w242) -> (x = y?=w252:bool)
          }
        }
      }
    }
    frame 3 {
      n128 = case shown="\"L\", Default" w298 {
        tunnel: w297 -> [w300 w354]
        frame "L", Default {
          # "Raise the elevator up 2.5 ft"
          # "Turn Left 90 degrees (in place)"
          # "Drive forward 15 ft"
          # "One possible bug that we might encounter is that the encoder won't reset the distance variables between movement actions.\nAlso, all numerical constants used for moving need to be finalized."
          # "Turn Left 90 degrees (in place)"
          # "Drive forward until past the switch (should be 20 ft)"
          n129 = call <vilib>:"WPI_RobotDriveRefNum Registry Get.vi"("refnum name"="Left and Right Motors") -> ("RobotDriveDevRef"=w307:T4)  [unwired: 1 in, 9 out]
          n130 = call <vilib>:"Get L&R Motor Encoder Outputs.vi"("Encoder Input in"=w300) -> ("Distance R"=w299:dbl)  [unwired: 5 in, 5 out]
          n131 = while {
            tunnel: w299 -> [w351]
            shift-right: [w346] -> w306
            shift-left: w307 -> [w347]
            tunnel: [w345] -> w305
            stop <- w352 stop-if-true
            w345 = "RobotDrive Motors" ("Name")
            n132 = call <vilib>:"WPI_RobotDriveTankDrive.vi"("Right axis value"=0.5 ("X axis value"), "Left axis value"=0.5 ("X axis value"), "RobotDriveDevRef"=w347) -> ("Motor Values"=w349:dbl[], "RobotDriveDevRef"=w350:T4)  [unwired: 6 in, 1 out]
            n133 = Equal?(x=240, y=w351) -> (x = y?=w352:bool)
            n134 = call-poly <vilib>:"NT Write Value.vi"("Numeric Array"=w349, "Name"=w345) -> ()  [unwired: 9 in, 1 out]
            n135 = call <vilib>:"WPI_RobotDriveDelayAndUpdateSafety.vi"("Delay (s)"=0.05, "RobotDriveDevRef"=w350) -> ("RobotDriveDevRef 2"=w346:T4)  [unwired: 8 in, 1 out]
          }
          n136 = while {
            shift-right: [w336] -> w303
            shift-left: w306 -> [w337]
            tunnel: [w332] -> w304
            tunnel: w305 -> [w332]
            tunnel: w299 -> [w331]
            stop <- w341 stop-if-true
            n137 = call <vilib>:"WPI_RobotDriveTankDrive.vi"("Right axis value"=0.5 ("X axis value"), "Left axis value"=-0.5 ("X axis value"), "RobotDriveDevRef"=w337) -> ("Motor Values"=w339:dbl[], "RobotDriveDevRef"=w340:T4)  [unwired: 6 in, 1 out]
            n138 = call-poly <vilib>:"NT Write Value.vi"("Numeric Array"=w339, "Name"=w332) -> ()  [unwired: 9 in, 1 out]
            n139 = call <vilib>:"WPI_RobotDriveDelayAndUpdateSafety.vi"("Delay (s)"=0.05, "RobotDriveDevRef"=w340) -> ("RobotDriveDevRef 2"=w336:T4)  [unwired: 8 in, 1 out]
            n140 = Equal?(x=19, y=w331) -> (x = y?=w341:bool)
          }
          n141 = while {
            tunnel: w299 -> [w329]
            shift-right: [w324] -> w301
            shift-left: w303 -> [w325]
            tunnel: [w320] -> w302
            tunnel: w304 -> [w320]
            stop <- w330 stop-if-true
            n142 = call <vilib>:"WPI_RobotDriveTankDrive.vi"("Right axis value"=0.5 ("X axis value"), "Left axis value"=0.5 ("X axis value"), "RobotDriveDevRef"=w325) -> ("Motor Values"=w327:dbl[], "RobotDriveDevRef"=w328:T4)  [unwired: 6 in, 1 out]
            n143 = call-poly <vilib>:"NT Write Value.vi"("Numeric Array"=w327, "Name"=w320) -> ()  [unwired: 9 in, 1 out]
            n144 = call <vilib>:"WPI_RobotDriveDelayAndUpdateSafety.vi"("Delay (s)"=0.05, "RobotDriveDevRef"=w328) -> ("RobotDriveDevRef 2"=w324:T4)  [unwired: 8 in, 1 out]
            n145 = Equal?(x=180, y=w329) -> (x = y?=w330:bool)
          }
          n146 = while {
            shift-right: [w314] -> _
            shift-left: w301 -> [w315]
            tunnel: w302 -> [w310]
            tunnel: w299 -> [w309]
            stop <- w319 stop-if-true
            n147 = call <vilib>:"WPI_RobotDriveTankDrive.vi"("Right axis value"=0.5 ("X axis value"), "Left axis value"=-0.5 ("X axis value"), "RobotDriveDevRef"=w315) -> ("Motor Values"=w317:dbl[], "RobotDriveDevRef"=w318:T4)  [unwired: 6 in, 1 out]
            n148 = call-poly <vilib>:"NT Write Value.vi"("Numeric Array"=w317, "Name"=w310) -> ()  [unwired: 9 in, 1 out]
            n149 = call <vilib>:"WPI_RobotDriveDelayAndUpdateSafety.vi"("Delay (s)"=0.05, "RobotDriveDevRef"=w318) -> ("RobotDriveDevRef 2"=w314:T4)  [unwired: 8 in, 1 out]
            n150 = Equal?(x=19, y=w309) -> (x = y?=w319:bool)
          }
        }
        frame "R" {
          # "Raise the elevator up 2.5 ft"
          # "Turn Left 90 degrees (in place)"
          # "Drive forward 4.5 ft"
          # "One possible bug that we might encounter is that the encoder won't reset the distance variables between movement actions.\nAlso, all numerical constants used for moving need to be finalized."
          # "Turn Left 90 degrees (in place)"
          # "Drive forward until past the switch (should be 20 ft)"
          n151 = call <vilib>:"WPI_RobotDriveRefNum Registry Get.vi"("refnum name"="Left and Right Motors") -> ("RobotDriveDevRef"=w361:T4)  [unwired: 1 in, 9 out]
          n152 = call <vilib>:"Get L&R Motor Encoder Outputs.vi"("Encoder Input in"=w354) -> ("Distance R"=w353:dbl)  [unwired: 5 in, 5 out]
          n153 = while {
            tunnel: w353 -> [w405]
            shift-right: [w400] -> w360
            shift-left: w361 -> [w401]
            tunnel: [w399] -> w359
            stop <- w406 stop-if-true
            w399 = "RobotDrive Motors" ("Name")
            n154 = call <vilib>:"WPI_RobotDriveTankDrive.vi"("Right axis value"=0.5 ("X axis value"), "Left axis value"=0.5 ("X axis value"), "RobotDriveDevRef"=w401) -> ("Motor Values"=w403:dbl[], "RobotDriveDevRef"=w404:T4)  [unwired: 6 in, 1 out]
            n155 = call-poly <vilib>:"NT Write Value.vi"("Numeric Array"=w403, "Name"=w399) -> ()  [unwired: 9 in, 1 out]
            n156 = call <vilib>:"WPI_RobotDriveDelayAndUpdateSafety.vi"("Delay (s)"=0.05, "RobotDriveDevRef"=w404) -> ("RobotDriveDevRef 2"=w400:T4)  [unwired: 8 in, 1 out]
            n157 = Equal?(x=240, y=w405) -> (x = y?=w406:bool)
          }
          n158 = while {
            shift-right: [w390] -> w357
            shift-left: w360 -> [w391]
            tunnel: [w386] -> w358
            tunnel: w359 -> [w386]
            tunnel: w353 -> [w385]
            stop <- w395 stop-if-true
            n159 = call <vilib>:"WPI_RobotDriveTankDrive.vi"("Right axis value"=0.5 ("X axis value"), "Left axis value"=-0.5 ("X axis value"), "RobotDriveDevRef"=w391) -> ("Motor Values"=w393:dbl[], "RobotDriveDevRef"=w394:T4)  [unwired: 6 in, 1 out]
            n160 = call-poly <vilib>:"NT Write Value.vi"("Numeric Array"=w393, "Name"=w386) -> ()  [unwired: 9 in, 1 out]
            n161 = call <vilib>:"WPI_RobotDriveDelayAndUpdateSafety.vi"("Delay (s)"=0.05, "RobotDriveDevRef"=w394) -> ("RobotDriveDevRef 2"=w390:T4)  [unwired: 8 in, 1 out]
            n162 = Equal?(x=19, y=w385) -> (x = y?=w395:bool)
          }
          n163 = while {
            tunnel: w353 -> [w383]
            shift-right: [w378] -> w355
            shift-left: w357 -> [w379]
            tunnel: [w374] -> w356
            tunnel: w358 -> [w374]
            stop <- w384 stop-if-true
            n164 = call <vilib>:"WPI_RobotDriveTankDrive.vi"("Right axis value"=0.5 ("X axis value"), "Left axis value"=0.5 ("X axis value"), "RobotDriveDevRef"=w379) -> ("Motor Values"=w381:dbl[], "RobotDriveDevRef"=w382:T4)  [unwired: 6 in, 1 out]
            n165 = call-poly <vilib>:"NT Write Value.vi"("Numeric Array"=w381, "Name"=w374) -> ()  [unwired: 9 in, 1 out]
            n166 = call <vilib>:"WPI_RobotDriveDelayAndUpdateSafety.vi"("Delay (s)"=0.05, "RobotDriveDevRef"=w382) -> ("RobotDriveDevRef 2"=w378:T4)  [unwired: 8 in, 1 out]
            n167 = Equal?(x=54, y=w383) -> (x = y?=w384:bool)
          }
          n168 = while {
            shift-right: [w368] -> _
            shift-left: w355 -> [w369]
            tunnel: w356 -> [w364]
            tunnel: w353 -> [w363]
            stop <- w373 stop-if-true
            n169 = call <vilib>:"WPI_RobotDriveTankDrive.vi"("Right axis value"=0.5 ("X axis value"), "Left axis value"=-0.5 ("X axis value"), "RobotDriveDevRef"=w369) -> ("Motor Values"=w371:dbl[], "RobotDriveDevRef"=w372:T4)  [unwired: 6 in, 1 out]
            n170 = call-poly <vilib>:"NT Write Value.vi"("Numeric Array"=w371, "Name"=w364) -> ()  [unwired: 9 in, 1 out]
            n171 = call <vilib>:"WPI_RobotDriveDelayAndUpdateSafety.vi"("Delay (s)"=0.05, "RobotDriveDevRef"=w372) -> ("RobotDriveDevRef 2"=w368:T4)  [unwired: 8 in, 1 out]
            n172 = Equal?(x=19, y=w363) -> (x = y?=w373:bool)
          }
        }
      }
    }
  }
  n173 = call <vilib>:"Get L&R Motor Encoder Outputs.vi"("Encoder Input in"="Encoder Input 2") -> ("Direction L"=→"Direction L 2":bool, "Distance L"=→"Distance L 2":dbl, "Direction R"=→"Direction L 2":bool, "Distance R"=→"Distance R 2":dbl, "Rate L"=→"Rate L 2":dbl, "Rate R"=→"Rate R 2":dbl)  [unwired: 5 in]
